vi "Aquire Continous Digital Port State.vi"() -> ()   [LabVIEW 2020]
uses:
  <instrlib>/BDAQ-6104/Examples/Read Single Digital Channel.vi
  <instrlib>/BDAQ-6104/BDAQ-6104.lvlib
panel:
  in  "Pin Direction":T1(array[cluster])
  out "Pin State":bool
  in  "stop":bool
  in  "VISA resource name":refnum<visa-resource-name>
  # "Continuously read the state of the spcified\ndigital pin until the user hits the STOP button."
  # "Input"
  # "Output"
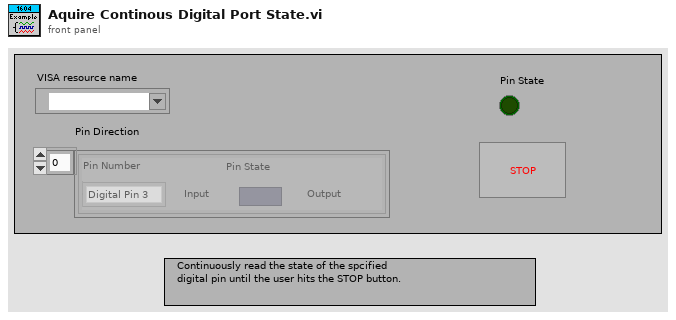
[diagram p1: front panel]
types:
  T1 = cluster{"Pin Number":enum16{"Digital Pin 0", "Digital Pin 1", "Digital Pin 2", "Digital Pin 3"}, "Pin State":bool}[]
  T2 = cluster{"Pin Number":enum16{"Digital Pin 0", "Digital Pin 1", "Digital Pin 2", "Digital Pin 3"}, "Pin State":bool}
  T3 = enum16{"Digital Pin 0", "Digital Pin 1", "Digital Pin 2", "Digital Pin 3"}
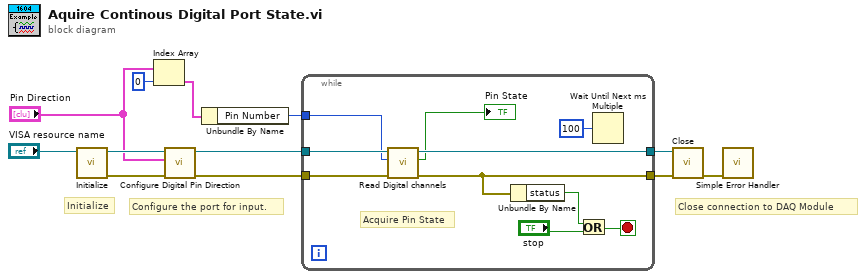
[diagram p0: block diagram]
diagram:
  # "Close connection to DAQ Module"
  # "Configure the port for input."
  # "Initialize"
  n1 = call <instrlib>:"Initialize.vi"("VISA resource name"="VISA resource name") -> ("error out"=w7:errorcluster, "VISA resource name out"=w8:refnum<visa-resource-name>)  [unwired: 9 in]
  n2 = Index Array(array="Pin Direction", index=0) -> (element=w2:T2)
  n3 = call <instrlib>:"Configure Digital Pin Direction.vi"("error in (no error)"=w7, "Pin Direction"="Pin Direction", "VISA resource name"=w8) -> ("error in (no error) 2"=w6:errorcluster, "VISA resource name 2"=w5:refnum<visa-resource-name>)  [unwired: 7 in]
  n4 = Unbundle By Name(w2) -> ("Pin Number"=w1:T3)
  n5 = while {
    tunnel: w5 -> [w21]
    tunnel: w6 -> [w20]
    tunnel: [w19] -> w10
    tunnel: [w15] -> w11
    tunnel: w1 -> [w13]
    stop <- w18 stop-if-true
    # "Acquire Pin State"
    n6 = call-poly <instrlib>:"Read Digital channels.vi"("error in (no error)"=w20, "Pin Number"=w13, "VISA resource name"=w21) -> ("error out"=w19:errorcluster, "Pin State"=→"Pin State":bool, "VISA resource name out"=w15:refnum<visa-resource-name>)  [unwired: 6 in]
    n7 = Unbundle By Name(w19) -> ("status"=w16:bool)
    n8 = Or(x=w16, y="stop") -> (x .or. y?=w18:bool)
    n9 = Wait Until Next ms Multiple(millisecond multiple=u32 100) -> ()  [unwired: 1 out]
  }
  n10 = call <instrlib>:"Close.vi"("error in (no error)"=w10, "VISA resource name"=w11) -> ("error out"=w9:errorcluster)  [unwired: 9 in]
  n11 = call <vilib>:"Simple Error Handler.vi"("error in (no error)"=w9) -> ()  [unwired: 4 in, 5 out]
